vi "Find By Team Number.vi"(10 "Team Number":u16) -> (2 "Found?":bool, 3 "Team Data":T1)   [LabVIEW 2013]
uses:
  Team Data.ctl
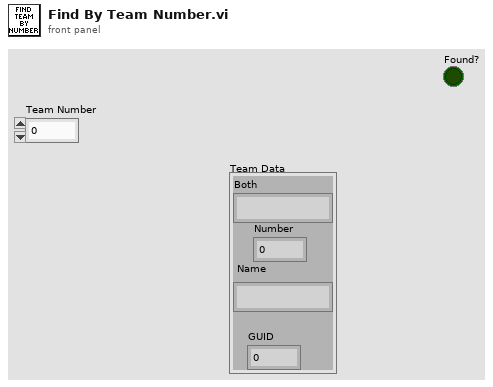
[diagram p1: front panel]
types:
  T1 = typedef "Team Data.ctl" = cluster{"Both":string, "Name":string, "GUID":u16, "Number":u16}
  T2 = enum16{"Get Teams", "Add Team", "Modify Team", "Clear All Teams", "Force Add Team", "Delete Team"}
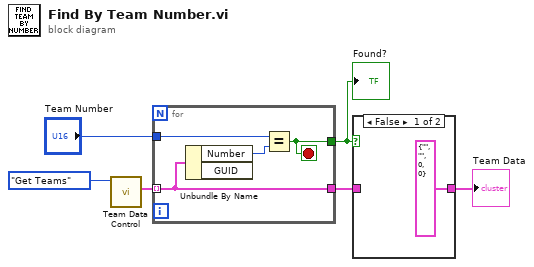
[diagram p0: block diagram]
diagram:
  n1 = call "Team Data Control.vi"("Mode"=T2."Get Teams") -> ("Team Array Out"=w1:T1[])  [unwired: 10 in]
  n2 = for {
    tunnel: w1 -> [w7] mode=indexing
    tunnel: "Team Number" -> [w9]
    tunnel: [w8] -> w5
    tunnel: [w7] -> w4
    stop <- w8 stop-if-true
    n3 = Unbundle By Name(w7) -> ("Number"=w10:u16)  [unwired: 1 out]
    n4 = Equal?(x=w9, y=w10) -> (x = y?=w8:bool)
  }
  "Found?" <- w5
  n5 = case shown="False" w5 {
    tunnel: [T1 {"Both"="", "Name"="", "GUID"=0, "Number"=0} ("Team Data") w12] -> w3
    tunnel: w4 -> [_ w12]
    frame False {
    }
    frame True {
    }
  }
  "Team Data" <- w3
